vi "HXG2_LOAD_Profile.vi"(8 "error in":errorcluster, 10 "Table":refnum<vi>, 11 "Programmer File":string) -> (0 "error out":errorcluster, 1 "Profile Save Path":path, 2 "Cell Values":string[][](array[string]), 3 "Headers":string[][](array[string]))   [LabVIEW 2012]
doc: "Load a profile's parameters to the table control"
uses:
  <vilib>/Utility/file.llb/Read From Spreadsheet File (string).vi
panel:
  out "Path to Profile":path
  # "C:\\Users\\AP5_Lab\\Documents\\HX_Calorimeter-SW\\trunk\\Other\\ProgrammerProfiles\\NewProfile.prof"
  # "C:\\Users\\AP5_Lab\\Documents\\HX_Calorimeter-SW\\trunk\\Other\\ProgrammerProfiles"
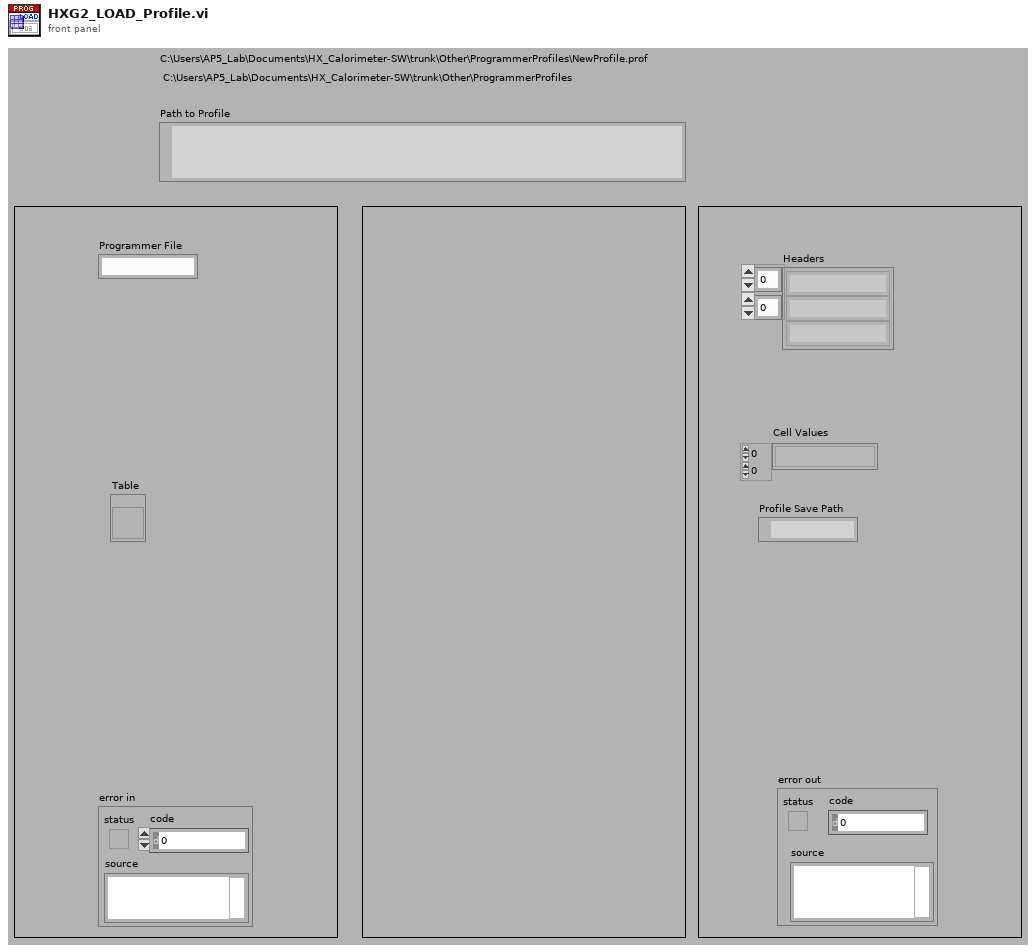
[diagram p1: front panel]
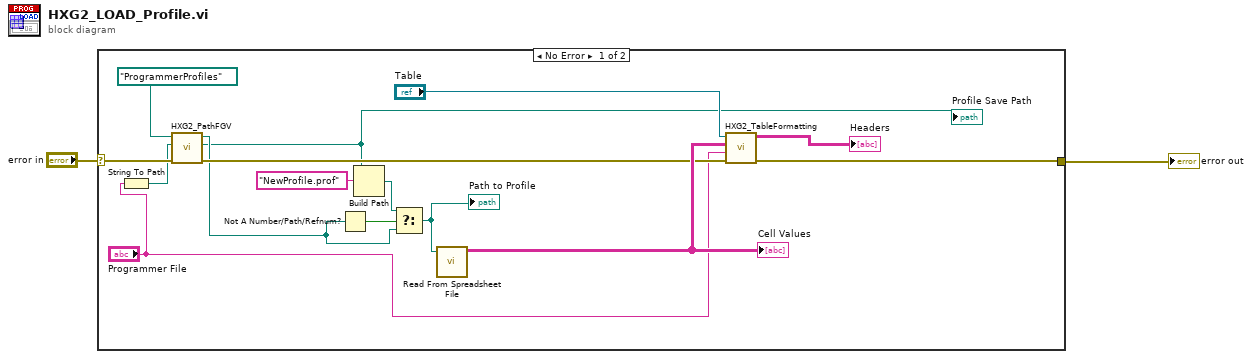
[diagram p0: block diagram]
diagram:
  n1 = case shown="No Error" "error in" {
    selector: "error in" -> [w9 w18]
    tunnel: [w13 w18] -> w2
    frame No Error {
      n2 = String To Path(string="Programmer File") -> (path=w6:path)
      n3 = call "HXG2_PathFGV.vi"("error in (no error)"=w9, "File Name"=w6, "Folder Name"=path "ProgrammerProfiles") -> ("error out"=w8:errorcluster, "Folder Path"=w4:path, "File path"=w5:path)  [unwired: 5 in, 1 out]
      "Profile Save Path" <- w4
      n4 = Not A Number/Path/Refnum?(number/path/refnum=w5) -> (NaN/Path/Refnum?=w17:bool)
      n5 = Build Path(base path=w4, name or relative path="NewProfile.prof") -> (appended path=w15:path)
      n6 = Select(t=w15, s=w17, f=w5) -> (s? t:f=w14:path)
      "Path to Profile" <- w14
      n7 = call-poly <vilib>:"Read From Spreadsheet File.vi"("file path (dialog if empty)"=w14) -> ("all rows"=w12:string[][])  [unwired: 6 in, 4 out]
      "Cell Values" <- w12
      n8 = call "HXG2_TableFormatting.vi"("error IO"=w8, "Programmer File"="Programmer File", "Data Array In"=w12, "Table Control"="Table") -> ("error out"=w13:errorcluster, "Headers"=→"Headers":string[][])  [unwired: 6 in]
    }
    frame Error {
    }
  }
  "error out" <- w2
